vi "fo_MWLQuery.vi"(8 "error in (no error)":errorcluster) -> (0 "error out":errorcluster, 1 "Cancel?":bool, 2 "Worklist":string[][](table), 3 "SelectedRow":string[](array[string]) caption="subarray")   [LabVIEW 2013, in "main.lvlib"]
uses:
  main.lvlib
  <vilib>/Utility/miscctls.llb/LVRowAndColumnTypeDef.ctl
  Controls/Enum Save Action Events.ctl
  Controls/SaveDataCluster.ctl
  <userlib>/_MGI/Error Handling/MGI Suppress Error Code/MGI Suppress Error Code (Scalar).vi
  <vilib>/Utility/cursorutil.llb/Set Cursor (Icon Pict).vi
panel:
  in  "TimeEnd":timestamp caption="End" format="%<%x>T"
  in  "TimeStart":timestamp caption="Start" format="%<%x>T"
  in  "SelectPatient":bool
  in  "Exit":bool
  in  "queryWorklist":bool
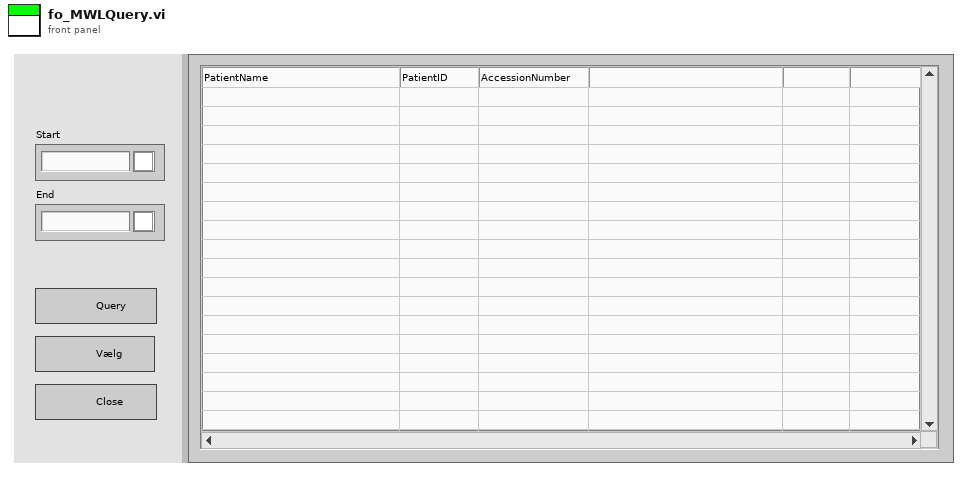
[diagram p1: front panel]
types:
  T1 = cluster{"port":i32, "AEtitle":string, "host":string, "remoteAE":string}
  T2 = typedef "main.lvlib/SaveDataCluster.ctl" = cluster{"HospInfo":cluster{"Name":string, "Address":string, "Department":string}, "Pressure":cluster{"Pressure":dbl}, "DataPath":cluster{"DataPath":path}, "ReportPath":cluster{"Path":path, "Name":string}, "DICOM Info WL":cluster{"port":i32, "AEtitle":string, "host":string, "remoteAE":string}, "DICOM Info PACS":cluster{"port":i32, "AEtitle":string, "host":string, "remoteAE":string}, "ArmCalcMethod":dbl, "itemTags":string[], "DicomEncoding":u16, "JournalType":u16, "General Settings":cluster{"Hyphenation":bool, "Language":u16, "CellStr1":string, "CellStr2":string}, "Dicom Tags":string[][], "BT Serial":cluster{"Serial Number":string, "Side":string, "Ignore?":bool}[], "BT License":cluster{"License":string, "Accepted Serials":string[]}}
  T3 = typedef "main.lvlib/Enum Save Action Events.ctl" = enum16{"LoadReportPath", "SaveReportPath", "Load Graph Path", "Save Graph Path", "LoadDataPath", "SaveDataPath", "Load Template Path", "Save Template Path", "Load PressureFactor", "Save PressureFactor", "Init", "Load Listbox", "Save Listbox", "LoadHospInfo", "SaveHospInfo", "Load DICOM Activation", "Save DICOM Activation", "LoadDICOMInfoWL", "SaveDICOMInfoWL", "LoadDICOMInfoPACS", "SaveDICOMInfoPACS", "Load ArmCalcMethod", "Save ArmCalcMethod", "LoadItemTags", "SaveItemTags", "LoadDICOMEncoding", "SaveDICOMEncoding", "LoadJournalType", "SaveJournalType", "LoadAcqFilterType", "SaveAcqFilterType", "Load Sequence", "Save Sequence", "Load Acquisition Mode", "Save Acquisition Mode", "Load General Settings", "Save General Settings", "Load Language", "Save Language", "Load Dicom Tags", "Save Dicom Tags", "Load BT Serial", "Save BT Serial", "Load BT License", "Save BT License"}
  T4 = typedef "LVRowAndColumnTypeDef.ctl" = cluster{"Row":i32, "Column":i32}
  T5 = typedef "LVDateTimeRec.ctl" = cluster{"fractional second":dbl, "second":i32, "minute":i32, "hour":i32, "day of month":i32, "month":i32, "year":i32, "day of week":i32, "day of year":i32, "DST":i32}
  T6 = cluster{"TimeStart":timestamp, "TimeEnd":timestamp}
  T7 = typedef "LVPoint32TypeDef.ctl" = cluster{"Horizontal":i32, "Vertical":i32}
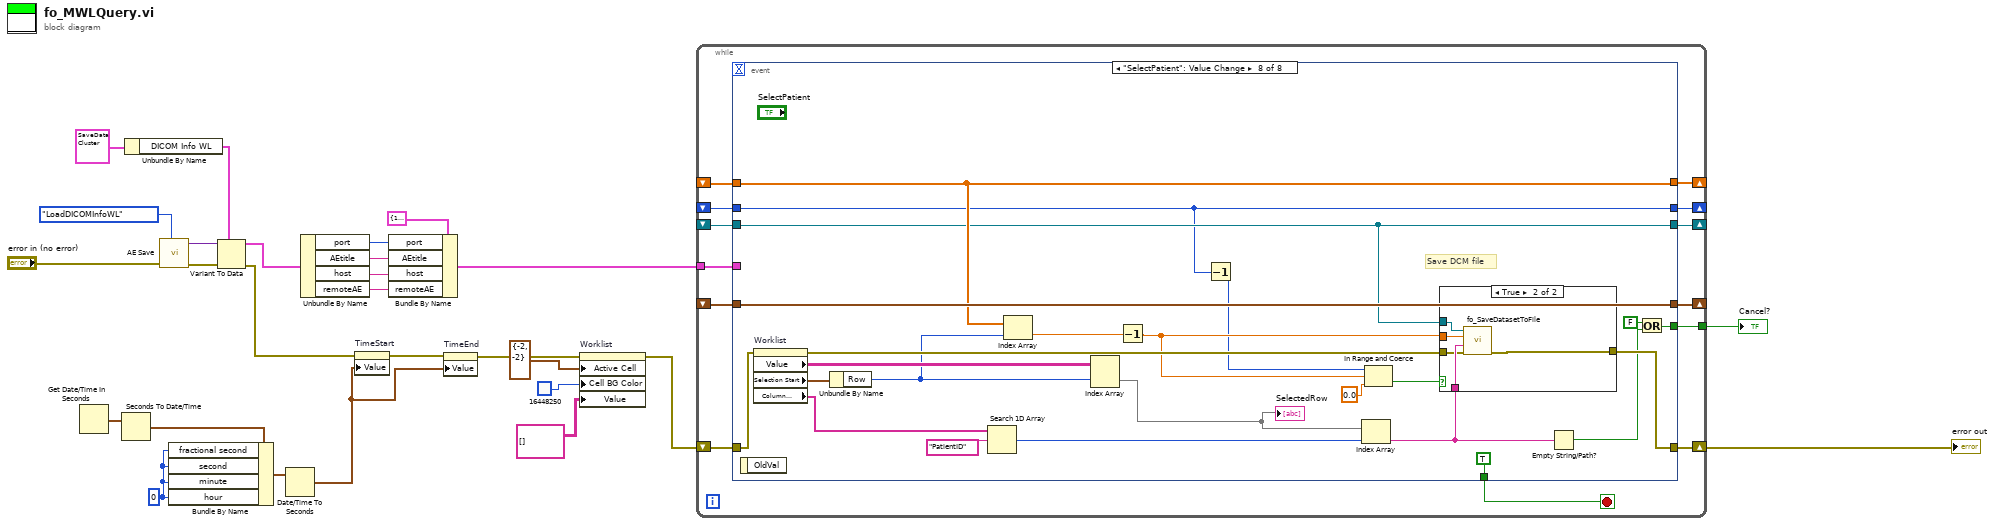
[diagram p0: block diagram]
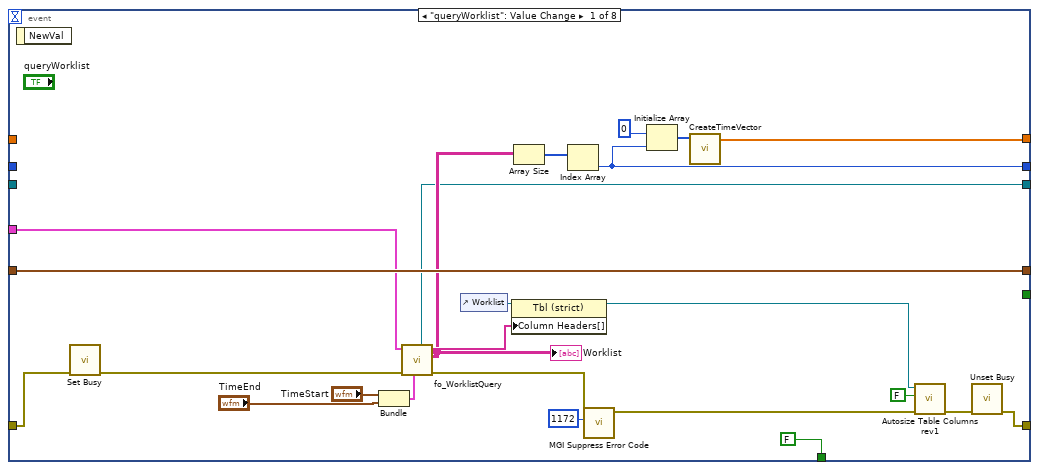
[diagram p2: hidden frame]
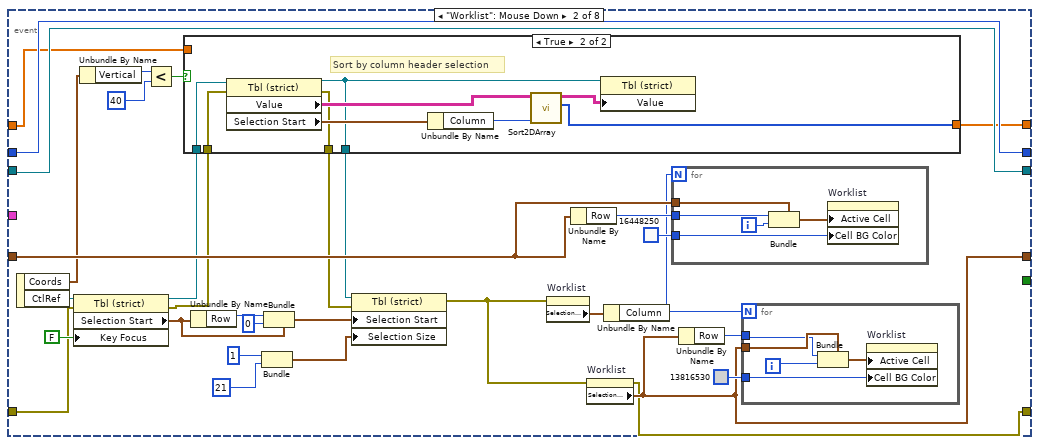
[diagram p3: hidden frame]
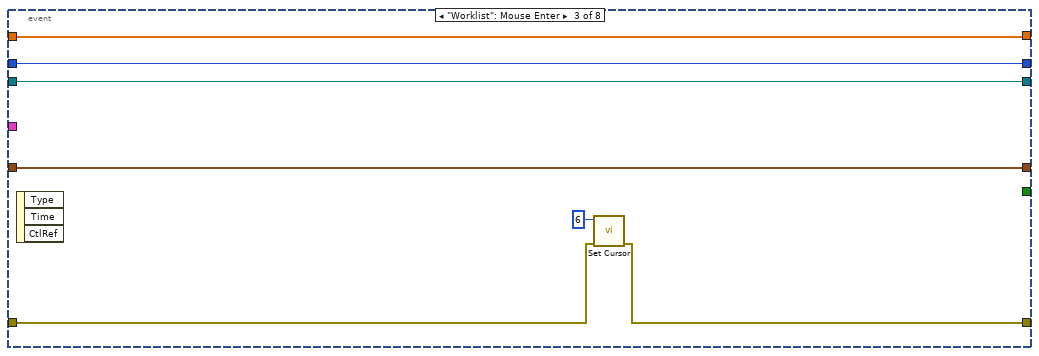
[diagram p5: hidden frame]
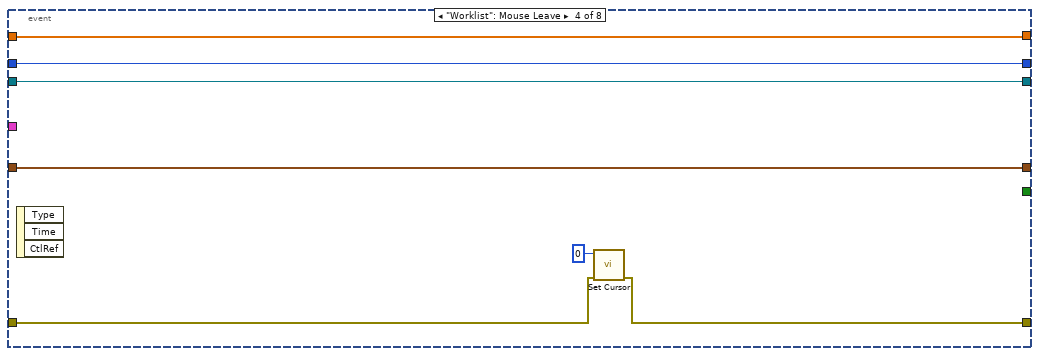
[diagram p6: hidden frame]
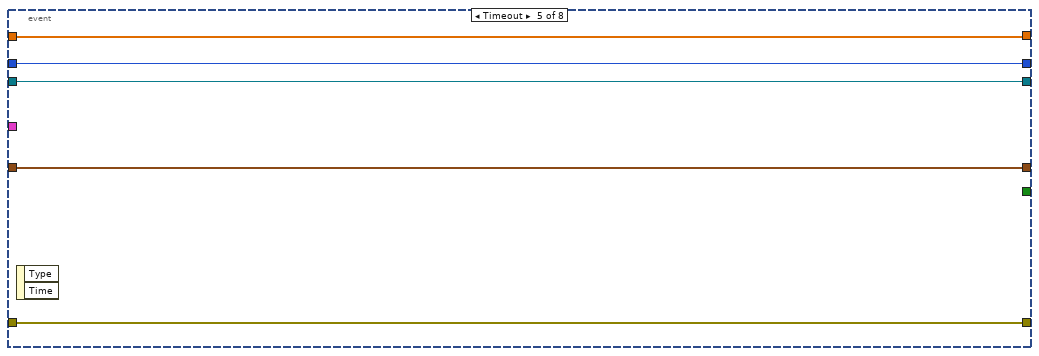
[diagram p7: hidden frame]
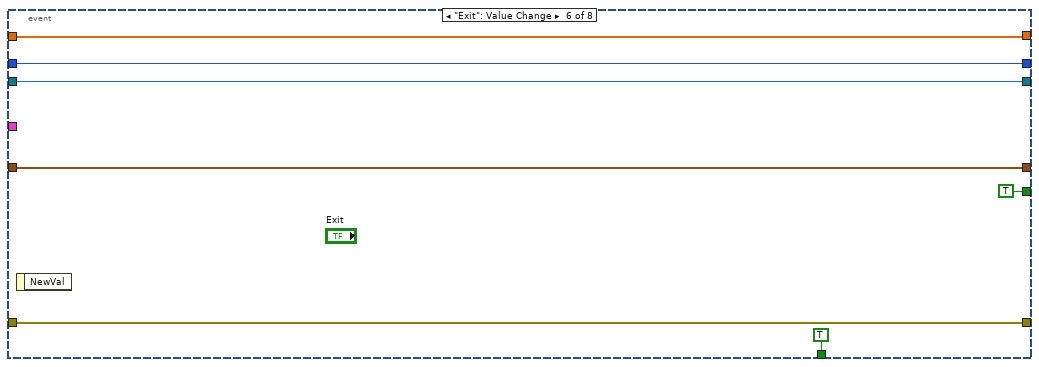
[diagram p8: hidden frame]
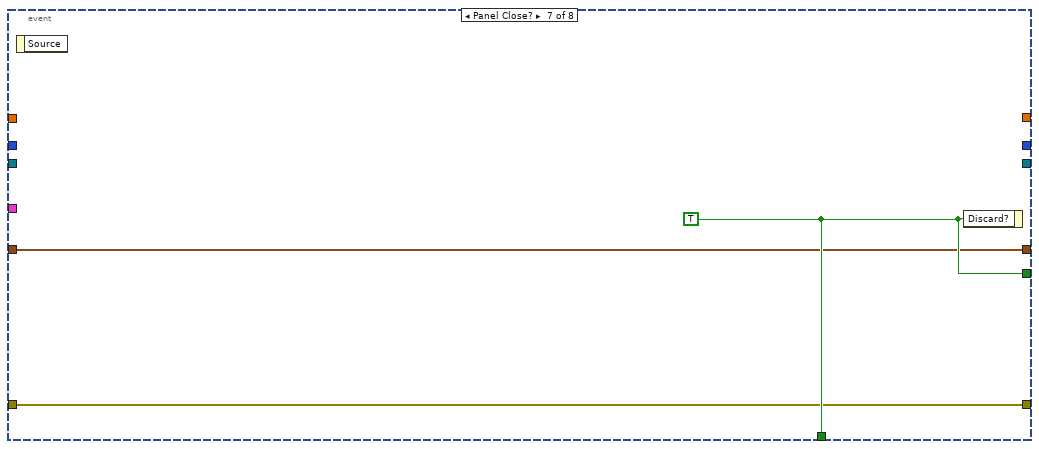
[diagram p9: hidden frame]
diagram:
  w4 = 0 ("hour")
  n1 = Get Date/Time In Seconds() -> (seconds since 1Jan1904=w3:timestamp)
  n2 = Seconds To Date/Time(time stamp (now)=w3) -> (date time rec=w5:T5)  [unwired: 1 in]
  n3 = Unbundle By Name(T2 {"HospInfo"={"Name"="", "Address"="", "Department"=""}, "Pressure"={"Pressure"=0.0}, "DataPath"={"DataPath"=path ""}, "ReportPath"={"Path"=path "", "Name"=""}, "DICOM Info WL"={"port"=0, "AEtitle"="", "host"="", "remoteAE"=""}, "DICOM Info PACS"={"port"=0, "AEtitle"="", "host"="", "remoteAE"=""}, "ArmCalcMethod"=0.0, "itemTags"=[], "DicomEncoding"=0, "JournalType"=0, "General Settings"={"Hyphenation"=FALSE, "Language"=0, "CellStr1"="", "CellStr2"=""}, "Dicom Tags"=[], "BT Serial"=[], "BT License"={"License"="", "Accepted Serials"=[]}} ("Data")) -> ("DICOM Info WL"=w17:T1)
  n4 = call "AE Save.vi"("error in (no error)"="error in (no error)", "Action"=Enum_Save_Action_Events."LoadDICOMInfoWL") -> ("error out"=w18:errorcluster, "Anything"=w22:variant)  [unwired: 7 in]
  n5 = Bundle By Name(cluster=w5, "fractional second"=w4, "second"=w4, "minute"=w4, "hour"=w4) -> (w2:T5)
  n6 = Variant To Data(error in=w18, type=w17, Variant=w22) -> (data=w20:T1, error out=w15:errorcluster)
  n7 = Date/Time To Seconds(2:w2) -> (0:w1:timestamp)  [unwired: 1 in]
  n8 = Unbundle By Name(w20) -> ("port"=w10:i32, "AEtitle"=w9:string, "host"=w8:string, "remoteAE"=w7:string)
  n9 = property on="TimeStart" class="AbsTime (strict)"(error in=w15, "Value"=w1) -> (error out=w14:errorcluster)  [unwired: 1 in, 1 out]
  n10 = Bundle By Name(cluster=T1 {"port"=1234, "AEtitle"="PSEUDO", "host"="OFFIS", "remoteAE"="127.0.0.1"} ("ServerInfo"), "port"=w10, "AEtitle"=w9, "host"=w8, "remoteAE"=w7) -> (w6:T1)
  n11 = property on="TimeEnd" class="AbsTime (strict)"(error in=w14, "Value"=w1) -> (error out=w13:errorcluster)  [unwired: 1 in, 1 out]
  n12 = property on="Worklist" class="Tbl (strict)"(error in=w13, "Active Cell"=T4 {"Row"=-2, "Column"=-2} ("Active Cell:Active Cell"), "Cell BG Color"=u32 16448250, "Value"=string[][] [] ("Worklist")) -> (error out=w25:errorcluster)  [unwired: 1 in, 1 out]
  n13 = while {
    shift-right: [w39] -> _
    shift-left: _ -> [w38]
    shift-right: [w36] -> w16
    shift-left: w25 -> [w37]
    shift-right: [w35] -> _
    shift-left: _ -> [w34]
    shift-right: [w33] -> _
    shift-left: _ -> [w32]
    shift-right: [w31] -> _
    shift-left: _ -> [w30]
    tunnel: [w29] -> w12
    tunnel: w6 -> [w28]
    stop <- w40 stop-if-true
    n14 = event shown="[7] \"SelectPatient\": Value Change" {
      selector: _ -> [_ _ _ _ _ _ _ _]
      dyn-events: _ -> [_ _ _ _ _ _ _ _]
      timeout: _ -> [_ _ _ _ _ _ _ _]
      tunnel: [FALSE _ _ _ _ TRUE w146 TRUE] -> w40
      tunnel: [w60 w91 w123 w130 w136 w142 w144 w169] -> w39
      tunnel: w38 -> [w60 w90 w123 w130 w136 w142 w144 w169]
      tunnel: w37 -> [w59 w79 w122 w129 w135 w141 w145 w167]
      tunnel: [w58 w78 w121 w128 w135 w141 w145 w165] -> w36
      tunnel: [w41 w77 w120 w127 w134 w140 _ w149] -> w35
      tunnel: w34 -> [_ w77 w120 w127 w134 w140 _ w149]
      tunnel: [w46 w76 w119 w126 w133 w139 _ w148] -> w33
      tunnel: w32 -> [_ w76 w119 w126 w133 w139 _ w148]
      tunnel: [w50 w67 w118 w125 w132 w138 _ w157] -> w31
      tunnel: w30 -> [_ w66 w118 w125 w132 w138 _ w157]
      tunnel: [_ _ _ _ _ TRUE w146 w152] -> w29
      tunnel: w28 -> [w44 _ _ _ _ _ _ _]
      event "queryWorklist": Value Change {
        n15 = event-data() -> ()  [unwired: 1 in, 1 out]
        n16 = call <vilib>:"Set Busy.vi"("error in (no error)"=w59) -> ("error out"=w43:errorcluster)  [unwired: 9 in, 1 out]
        n17 = Bundle("TimeStart"="TimeStart", "TimeEnd"="TimeEnd") -> (w45:T6)  [unwired: 1 in]
        n18 = call "fo_WorklistQuery.vi"("DateRange"=w45, "error in (no error)"=w43, "ServerInfo"=w44) -> ("error out"=w61:errorcluster, "Result Array"=w48:string[][], "Tags"=w49:string[], "Results"=w41:refnum<k24>)  [unwired: 5 in]
        "Worklist" <- w48
        n19 = control-ref of="Worklist"() -> (w54:refnum<vi>)
        n20 = property class="Tbl (strict)"(reference=w54, "Column Headers[]"=w49) -> (reference out=w53:refnum<vi>)  [unwired: 1 in, 1 out]
        n21 = Array Size(array=w48) -> (size(s)=w47:i32[])
        n22 = Index Array(array=w47) -> (element=w46:i32)  [unwired: 1 in]
        n23 = call-poly <userlib>:"MGI Suppress Error Code.vi"("Error Code"=1172, "Error In"=w61) -> ("Error Out"=w42:errorcluster)  [unwired: 4 in, 1 out]
        n24 = Initialize Array(0 ("dimension size"), w46) -> (w51:i32[])
        n25 = call "CreateTimeVector.vi"("Array in"=w51) -> ("Array out"=w50:dbl[])  [unwired: 10 in]
        n26 = call "Autosize Table Columns rev1.vi"("error in (no error)"=w42, "Resize Table?"=FALSE, "Table Ref"=w53) -> ()  [unwired: 4 in, 1 out]
        n27 = call <vilib>:"Unset Busy.vi"("error in (no error)"=w42) -> ("error out"=w58:errorcluster)  [unwired: 10 in]
      }
      event "Worklist": Mouse Down {
        n28 = event-data() -> ("Coords"=w74:T7, "CtlRef"=w73:refnum<vi>)  [unwired: 1 in]
        n29 = property class="Tbl (strict)"(reference=w73, error in=w79, "Key Focus"=FALSE) -> (reference out=w68:refnum<vi>, error out=w65:errorcluster, "Selection Start"=w88:T4)
        n30 = Unbundle By Name(w74) -> ("Vertical"=w72:i32)
        n31 = Less?(x=w72, y=40) -> (x < y?=w70:bool)
        n32 = case shown="True" w70 {
          tunnel: [w98 w103] -> w69
          tunnel: w68 -> [w98 w102]
          tunnel: [w97 w101] -> w67
          tunnel: w66 -> [w97 _]
          tunnel: w65 -> [w96 w100]
          tunnel: [w96 w99] -> w64
          frame False {
          }
          frame True {
            # "Sort by column header selection"
            n33 = property class="Tbl (strict)"(reference=w102, error in=w100) -> (reference out=w103:refnum<vi>, error out=w99:errorcluster, "Value"=w106:string[][], "Selection Start"=w107:T4)
            n34 = Unbundle By Name(w107) -> ("Column"=w105:i32)
            n35 = call "Sort2DArray.vi"("\"Sort on\" Col/Row indx (0)"=w105, "Array in"=w106) -> ("Sort indices"=w101:i32[], "Sorted Array"=w104:string[][])  [unwired: 7 in, 1 out]
            n36 = property class="Tbl (strict)"(reference=w103, "Value"=w104) -> ()  [unwired: 1 in, 2 out]
          }
        }
        n37 = Unbundle By Name(w88) -> ("Row"=w87:i32)
        n38 = Bundle(1, 21) -> (w83:cluster{i32, i32})  [unwired: 1 in]
        n39 = Bundle(cluster=w88, "Row"=w87, "Column"=0) -> (w84:T4)
        n40 = property class="Tbl (strict)"(reference=w69, error in=w64, "Selection Start"=w84, "Selection Size"=w83) -> (error out=w82:errorcluster)  [unwired: 1 out]
        n41 = property on="Worklist" class="Tbl (strict)"(error in=w82) -> ("Selection Size"=w81:T4)  [unwired: 1 in, 2 out]
        n42 = Unbundle By Name(w90) -> ("Row"=w93:i32)
        n43 = property on="Worklist" class="Tbl (strict)"(error in=w82) -> (error out=w78:errorcluster, "Selection Start"=w91:T4)  [unwired: 1 in, 1 out]
        n44 = Unbundle By Name(w81) -> ("Column"=w80:i32)
        n45 = for {
          N: w80 -> [_]
          tunnel: u32 16448250 -> [w112]
          tunnel: w90 -> [w111]
          tunnel: w93 -> [w110]
          i -> [w109]
          n46 = Bundle(cluster=w111, "Row"=w110, "Column"=w109) -> (w108:T4)
          n47 = property on="Worklist" class="Tbl (strict)"("Active Cell"=w108, "Cell BG Color"=w112) -> ()  [unwired: 2 in, 2 out]
        }
        n48 = Unbundle By Name(w91) -> ("Row"=w94:i32)
        n49 = for {
          N: w80 -> [_]
          tunnel: u32 13816530 -> [w117]
          tunnel: w91 -> [w116]
          tunnel: w94 -> [w115]
          i -> [w114]
          n50 = Bundle(cluster=w116, "Row"=w115, "Column"=w114) -> (w113:T4)
          n51 = property on="Worklist" class="Tbl (strict)"("Active Cell"=w113, "Cell BG Color"=w117) -> ()  [unwired: 2 in, 2 out]
        }
      }
      event "Worklist": Mouse Enter {
        n52 = event-data() -> ()  [unwired: 1 in, 3 out]
        n53 = call-poly <vilib>:"Set Cursor.vi"("error in (no error)"=w122, "icon"=u16 6) -> ("error out"=w121:errorcluster)  [unwired: 8 in, 1 out]
      }
      event "Worklist": Mouse Leave {
        n54 = event-data() -> ()  [unwired: 1 in, 3 out]
        n55 = call-poly <vilib>:"Set Cursor.vi"("error in (no error)"=w129, "icon"=u16 0) -> ("error out"=w128:errorcluster)  [unwired: 8 in, 1 out]
      }
      event Timeout {
        n56 = event-data() -> ()  [unwired: 1 in, 2 out]
      }
      event "Exit": Value Change {
        n57 = event-data() -> ()  [unwired: 1 in, 1 out]
      }
      event Panel Close? {
        w146 = TRUE ("Discard?")
        n58 = event-data() -> ()  [unwired: 1 in, 1 out]
        n59 = event-data("Discard?"=w146) -> ()  [unwired: 1 in, 1 out]
      }
      event "SelectPatient": Value Change {
        # "Save DCM file"
        n60 = event-data() -> ()  [unwired: 1 in, 1 out]
        n61 = property on="Worklist" class="Tbl (strict)"(error in=w167) -> (error out=w166:errorcluster, "Value"=w162:string[][], "Selection Start"=w170:T4, "Column Headers[]"=w158:string[])  [unwired: 1 in, 1 out]
        n62 = Unbundle By Name(w170) -> ("Row"=w156:i32)
        n63 = Search 1D Array(1D array=w158, element="PatientID") -> (index of element=w160:i32)  [unwired: 1 in]
        n64 = Index Array(array=w157, index=w156) -> (element=w154:dbl)
        n65 = Index Array(array=w162, index (row)=w156) -> (element=w159:string[])  [unwired: 1 in]
        "SelectedRow" <- w159
        n66 = Decrement(x=w154) -> (x-1=w155:dbl)
        n67 = Decrement(x=w148) -> (x-1=w147:i32)
        n68 = Index Array(array=w159, index=w160) -> (element=w153:string)
        n69 = In Range and Coerce(upper limit=w147, x=w155, lower limit=0.0) -> (In Range?=w163:bool)  [unwired: 1 out]
        n70 = case shown="True" w163 {
          tunnel: w166 -> [w171 w174]
          tunnel: [w171 w176] -> w165
          tunnel: w155 -> [_ w173]
          tunnel: w153 -> [_ w175]
          tunnel: w149 -> [_ w172]
          frame False {
          }
          frame True {
            n71 = call "fo_SaveDatasetToFile.vi"("error in (no error)"=w174, "patientID"=w175, "Dataset index"=w173, "Results"=w172) -> ("error out"=w176:errorcluster)  [unwired: 7 in]
          }
        }
        n72 = Empty String/Path?(string/path=w153) -> (empty?=w150:bool)
        n73 = Or(x=FALSE, y=w150) -> (x .or. y?=w152:bool)
      }
    }
  }
  "error out" <- w16
  "Cancel?" <- w12
